vi "Initialize Logger.vi"(8 "error in (no error)":errorcluster, 11 "Data Cluster OUT in":T1 {"Measurement Configuration"."Relative To" items=["Power sequence start", "Previous source start", "Previous source end"]; "Measurement Configuration"."Power line frequency" items=["50 Hz", "60 Hz"]; "Measurement Configuration"."Start Value" format="%#_6p"; "Measurement Configuration"."Transient Response" items=["Slow", "Normal", "Fast"]; "Measurement Configuration"."Sense Mode" items=["Local Sense", "Remote Sense"]; "Measurement Configuration"."Target Value" format="%#_6p"; "Measurement Configuration"."Source Mode" items=["DC Voltage", "DC Current"]; "Measurement Configuration"."Start Delay" format="%#_6p"; "Measurement Configuration"."Compliance Limit" format="%#_6p"; "Measurement Configuration"."Ramp Rate" format="%#_6p"}) -> (0 "error out":errorcluster, 3 "Data Cluster OUT out":T1 {"Measurement Configuration"."Relative To" items=["Power sequence start", "Previous source start", "Previous source end"]; "Measurement Configuration"."Power line frequency" items=["50 Hz", "60 Hz"]; "Measurement Configuration"."Start Value" format="%#_6p"; "Measurement Configuration"."Transient Response" items=["Slow", "Normal", "Fast"]; "Measurement Configuration"."Sense Mode" items=["Local Sense", "Remote Sense"]; "Measurement Configuration"."Target Value" format="%#_6p"; "Measurement Configuration"."Source Mode" items=["DC Voltage", "DC Current"]; "Measurement Configuration"."Start Delay" format="%#_6p"; "Measurement Configuration"."Compliance Limit" format="%#_6p"; "Measurement Configuration"."Ramp Rate" format="%#_6p"})   [LabVIEW 2024, in "devicePowerSequencerCoreLogic.lvlib"]
doc: "Create new log file ."
uses:
  devicePowerSequencerCoreLogic.lvlib
  controls/Data Cluster.ctl
  <vilib>/Plug-In SDKs/Clients/Session Management V1/Session Reservation/Session Reservation.lvclass
  <vilib>/Plug-In SDKs/Measurements/Measure Call Context/Measure Call Context.lvclass
  Measurement Configuration.ctl
  controls/Source Mode.ctl
  controls/Sense Mode.ctl
  controls/Relative To.ctl
  controls/Transient Response.ctl
  controls/Power line frequency.ctl
  Measurement Results.ctl
  controls/Channel Name.ctl
  controls/Software Flags.ctl
  controls/Ramp Configurations.ctl
  controls/Error Info.ctl
  controls/Measurements.ctl
  controls/Voltage and Current Measurements.ctl
  controls/Log Configurations.ctl
  dataLogger/dataLogger.lvlib
  Device Power Sequencer.lvlib
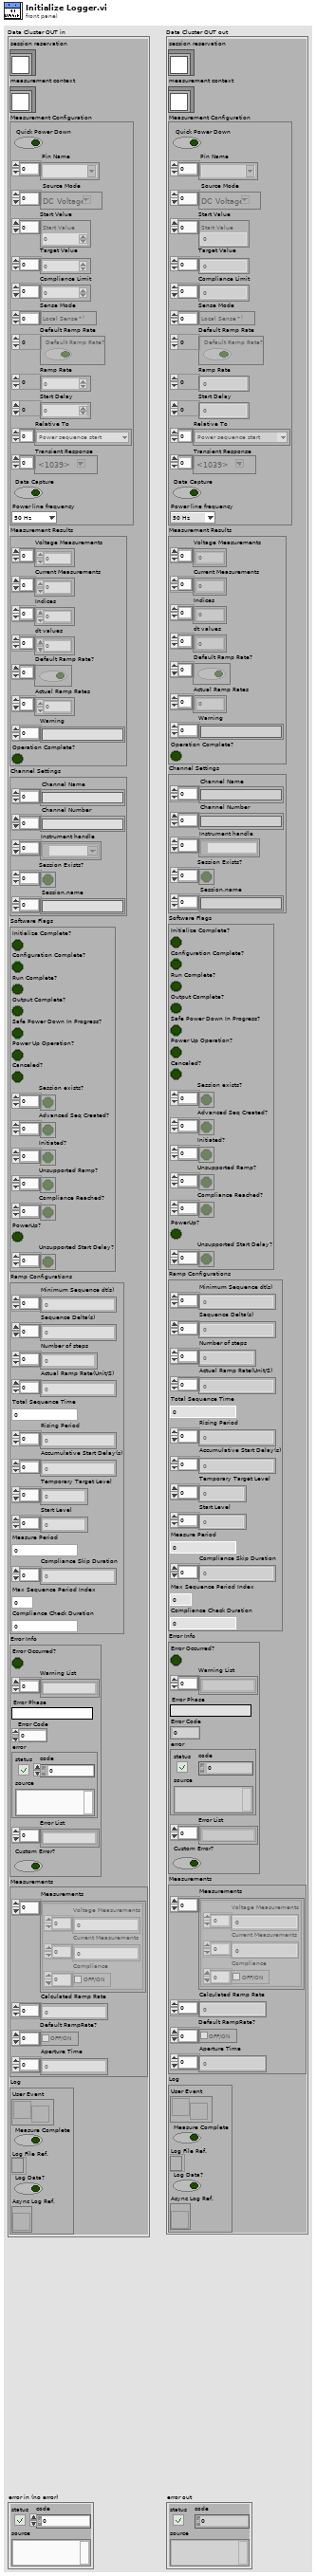
[diagram p1: front panel]
types:
  T1 = typedef "devicePowerSequencerCoreLogic.lvlib/Data Cluster.ctl" = cluster{"session reservation":refnum<class "Session Reservation.lvclass">, "measurement context":refnum<class "Measure Call Context.lvclass">, "Measurement Configuration":T2, "Measurement Results":T8, "Channel Settings":T9, "Software Flags":T10, "Ramp Configurations":T11, "Error Info":T12, "Measurements":T13, "Log":T15}
  T2 = typedef "Device Power Sequencer.lvlib/Measurement Configuration.ctl" = cluster{"Quick Power Down":bool, "Pin Name":string[], "Source Mode":T3[], "Start Value":dbl[], "Target Value":dbl[], "Compliance Limit":dbl[], "Sense Mode":T4[], "Default Ramp Rate":bool[], "Ramp Rate":dbl[], "Start Delay":dbl[], "Relative To":T5[], "Transient Response":T6[], "Data Capture":bool, "Power line frequency":T7}
  T3 = typedef "Device Power Sequencer.lvlib/Source Mode.ctl" = i32
  T4 = typedef "Device Power Sequencer.lvlib/Sense Mode.ctl" = i32
  T5 = typedef "Device Power Sequencer.lvlib/Relative To.ctl" = u32
  T6 = typedef "Device Power Sequencer.lvlib/Transient Response.ctl" = i32
  T7 = typedef "Device Power Sequencer.lvlib/Power line frequency.ctl" = u32
  T8 = typedef "Device Power Sequencer.lvlib/Measurement Results.ctl" = cluster{"Voltage Measurements":dbl[], "Current Measurements":dbl[], "Indices":i32[], "dt values":dbl[], "Default Ramp Rate?":bool[], "Actual Ramp Rates":dbl[], "Warning":string[], "Operation Complete?":bool}
  T9 = typedef "devicePowerSequencerCoreLogic.lvlib/Channel Name.ctl" = cluster{"Channel Name":string[], "Channel Number":string[], "Instrument handle":refnum<k15>[], "Session Exists?":bool[], "Session.name":string[]}
  T10 = typedef "devicePowerSequencerCoreLogic.lvlib/Software Flags.ctl" = cluster{"Initialize Complete?":bool, "Configuration Complete?":bool, "Run Complete?":bool, "Output Complete?":bool, "Safe Power Down In Progress?":bool, "Power Up Operation?":bool, "Canceled?":bool, "Session exists?":bool[], "Advanced Seq Created?":bool[], "Initiated?":bool[], "Unsupported Ramp?":bool[], "Compliance Reached?":bool[], "PowerUp?":bool, "Unsupported Start Delay?":bool[]}
  T11 = typedef "devicePowerSequencerCoreLogic.lvlib/Ramp Configurations.ctl" = cluster{"Minimum Sequence dt(s)":dbl[], "Sequence Delta(s)":dbl[], "Number of steps":i32[], "Actual Ramp Rate(Unit/S)":dbl[], "Total Sequence Time":dbl, "Rising Period":dbl[], "Accumulative Start Delay(s)":dbl[], "Temporary Target Level":dbl[], "Start Level":dbl[], "Measure Period":dbl, "Compliance Skip Duration":dbl[], "Max Sequence Period Index":i32, "Compliance Check Duration":dbl}
  T12 = typedef "devicePowerSequencerCoreLogic.lvlib/Error Info.ctl" = cluster{"Error Occurred?":bool, "Warning List":string[], "Error Phase":string, "Error Code":i32, "error":errorcluster, "Error List":string[], "Custom Error?":bool}
  T13 = typedef "devicePowerSequencerCoreLogic.lvlib/Measurements.ctl" = cluster{"Measurements":T14[], "Calculated Ramp Rate":dbl[], "Default RampRate?":bool[], "Aperture Time":dbl[]}
  T14 = typedef "devicePowerSequencerCoreLogic.lvlib/Voltage and Current Measurements.ctl" = cluster{"Voltage Measurements":dbl[], "Current Measurements":dbl[], "Compliance":bool[]}
  T15 = typedef "devicePowerSequencerCoreLogic.lvlib/Log Configurations.ctl" = cluster{"User Event":refnum<user-event>, "Measure Complete":bool, "Log File Ref.":refnum<file>, "Log Data?":bool, "Async Log Ref.":refnum<vi>}
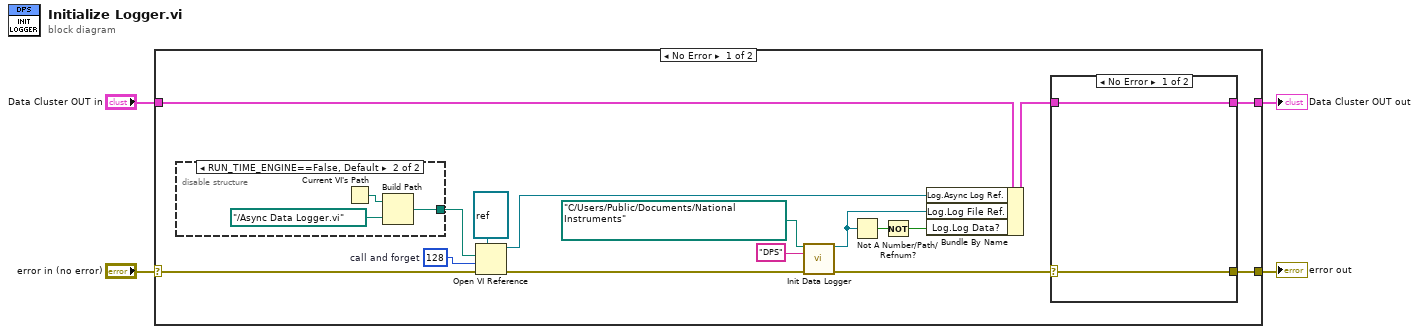
[diagram p0: block diagram]
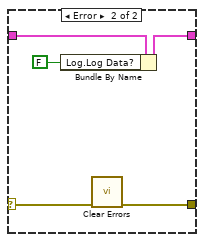
[diagram p2: hidden frame]
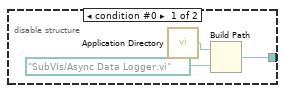
[diagram p3: hidden frame]
diagram:
  n1 = case shown="No Error" "error in (no error)" {
    selector: "error in (no error)" -> [w5 w34]
    tunnel: [w20 w34] -> w4
    tunnel: [w19 w35] -> w3
    tunnel: "Data Cluster OUT in" -> [w6 w35]
    frame No Error {
      w10 = 128  # call and forget
      n2 = disable-structure shown="RUN_TIME_ENGINE==False, Default" {
        disable-tunnel: [w28 w31] -> w12
        frame condition #0 {
          n3 = call <vilib>:"Application Directory.vi"() -> ("Application Directory"=w30:path)
          n4 = Build Path(base path=w30, name or relative path=path "SubVIs/Async Data Logger.vi") -> (appended path=w28:path)
        }
        frame condition #1 (active) {
          n5 = Current VI's Path() -> (path=w33:path)
          n6 = Build Path(base path=w33, name or relative path=path "../Async Data Logger.vi") -> (appended path=w31:path)
        }
      }
      n7 = Open VI Reference(type specifier VI Refnum (for type only)=refnum<vi> refnum, vi path=w12, options=w10, error in (no error)=w5) -> (vi reference=w16:refnum<vi>, error out=w11:errorcluster)  [unwired: 2 in]
      n8 = call "Init Data Logger.vi"("Log File Path"=path "C:/Users/Public/Documents/National Instruments", "Module"="DPS", "error in"=w11) -> ("Log File Ref. Out"=w14:refnum<file>, "error out"=w17:errorcluster)  [unwired: 10 in, 1 out]
      n9 = Not A Number/Path/Refnum?(number/path/refnum=w14) -> (NaN/Path/Refnum?=w13:bool)
      n10 = Not(x=w13) -> (.not. x?=w15:bool)
      n11 = Bundle By Name(cluster=w6, "Log.Async Log Ref."=w16, "Log.Log File Ref."=w14, "Log.Log Data?"=w15) -> (w18:T1)
      n12 = case shown="No Error" w17 {
        selector: w17 -> [w22 w26]
        tunnel: [w21 w25] -> w19
        tunnel: w18 -> [w21 w27]
        tunnel: [w22 w23] -> w20
        frame No Error {
        }
        frame Error {
          n13 = Bundle By Name(cluster=w27, "Log.Log Data?"=FALSE) -> (w25:T1)
          n14 = call <vilib>:"Clear Errors.vi"("error in (no error)"=w26) -> ("error out"=w23:errorcluster)  [unwired: 5 in, 1 out]
        }
      }
    }
    frame Error {
    }
  }
  "error out" <- w4
  "Data Cluster OUT out" <- w3
